vi "RSZVB Default Instrument Setup.vi"(8 "error in (no error)":errorcluster {"code" format="%.0x"}, 11 "VISA session":refnum<visa-resource-name>) -> (0 "error out":errorcluster {"code" format="%.0x"}, 3 "dup VISA session":refnum<visa-resource-name>)   [LabVIEW 2015]
doc: "This Utility VI sends a default command string to the instrument whenever a new VISA session is opened, or the instrument is reset. This VI is intended to be used as a subVI for the RSZVB Initialize and RSZVB Reset VI's. Altering this VI could cause these two VI's to operate incorrectly."
uses:
  _utility/RSZVB Global Data.vi
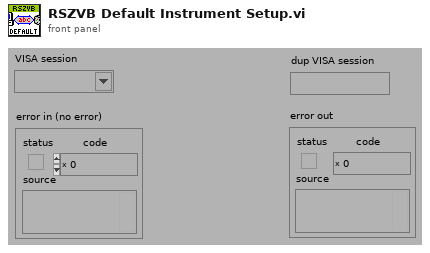
[diagram p1: front panel]
types:
  T1 = cluster{"Version Major":i32, "Version Minor":i32}
  T2 = cluster{"Error Checking (T: On)":bool, "Installed Options":string[], "Data Valid?":bool, "Ports":i32, "Model":string[], "Option Checking (T: On)":bool}[]
  T3 = cluster{"Error Checking (T: On)":bool, "Installed Options":string[], "Data Valid?":bool, "Ports":i32, "Model":string[], "Option Checking (T: On)":bool}
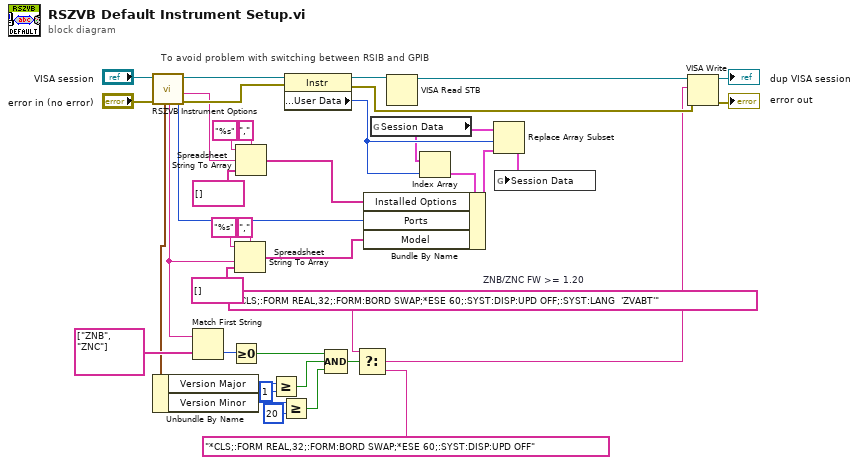
[diagram p0: block diagram]
diagram:
  w9 = "*CLS;:FORM REAL,32;:FORM:BORD SWAP;*ESE 60;:SYST:DISP:UPD OFF;:SYST:LANG  'ZVABT'"  # ZNB/ZNC FW >= 1.20
  # "To avoid problem with switching between RSIB and GPIB"
  n1 = call "RSZVB Instrument Options.vi"("error in (no error)"="error in (no error)", "VISA session"="VISA session") -> ("error out"=w31:errorcluster, "Options List"=w29:string, "dup VISA session"=w30:refnum<visa-resource-name>, "Ports"=w27:i32, "Model"=w17:string, "Version"=w7:T1)  [unwired: 3 in, 1 out]
  n2 = Unbundle By Name(w7) -> ("Version Major"=w3:i32, "Version Minor"=w6:i32)
  n3 = Match First String(2:string[] ["ZNB", "ZNC"] ("string array"), 3:w17) -> (0:w15:i32)  [unwired: 1 out]
  n4 = Greater Or Equal To 0?(x=w15) -> (x >= 0?=w11:bool)
  n5 = Spreadsheet String To Array(delimiter (Tab)=",", format string="%s", spreadsheet string=w17, array type (2D Dbl)=string[] []) -> (array=w23:string[])
  n6 = Spreadsheet String To Array(delimiter (Tab)=",", format string="%s", spreadsheet string=w29, array type (2D Dbl)=string[] []) -> (array=w28:string[])
  n7 = Greater Or Equal?(x=w3, y=1) -> (x >= y?=w2:bool)
  n8 = Greater Or Equal?(x=w6, y=20) -> (x >= y?=w1:bool)
  n9 = property class="Instr"(reference=w30, error in=w31) -> (reference out=w22:refnum<visa-resource-name>, error out=w20:errorcluster, "General Settings:User Data"=w39:u32)
  n10 = Compound Arithmetic op=AND(w11, w2, w1) -> (w10:bool)
  n11 = Select(t=w9, s=w10, f="*CLS;:FORM REAL,32;:FORM:BORD SWAP;*ESE 60;:SYST:DISP:UPD OFF" ("Default Setup String")) -> (s? t:f=w14:string)
  n12 = global read "RSZVB Global Data.vi" "Session Data"() -> (w35:T2)
  n13 = VISA Read STB(11:w22) -> (3:w21:refnum<visa-resource-name>)  [unwired: 1 in, 2 out]
  n14 = Index Array(array=w35, index=w39) -> (element=w38:T3)
  n15 = Bundle By Name(cluster=w38, "Installed Options"=w28, "Ports"=w27, "Model"=w23) -> (w37:T3)
  n16 = Replace Array Subset(array=w35, new element=w37, index=w39) -> (w36:T2)
  n17 = global write "RSZVB Global Data.vi" "Session Data"(w36) -> ()
  n18 = VISA Write(VISA resource name=w21, write buffer=w14, error in (no error)=w20) -> (VISA resource name out=→"dup VISA session":refnum<visa-resource-name>, error out=→"error out":errorcluster)  [unwired: 1 out]
